vi "PID Controller.vi"() -> ()   [LabVIEW 2014]
panel:
  in  "Sample/sec":i32(slide) scale=0.0..50.0
  out "?":bool
  out "SP Vs PV":cluster{dbl, dbl}(knob)={0.0, 20.65645025147849} scale=0.0..60.0
  in  "?":bool
  in  "I":dbl=0.5
  in  "D":dbl=0.2
  in  "P":dbl=0.56
  in  "Minimum":dbl
  in  "Maximum":dbl=60.0
  in  "Set Point":dbl(slide)=50.0 scale=0.0..60.0
  out "Waveform Chart":cluster{"Set Point":dbl, "output variable":dbl}(graph)={"Set Point"=49.70711297071129, "output variable"=49.707112970712004}
  # "PID Temperature Controlller"
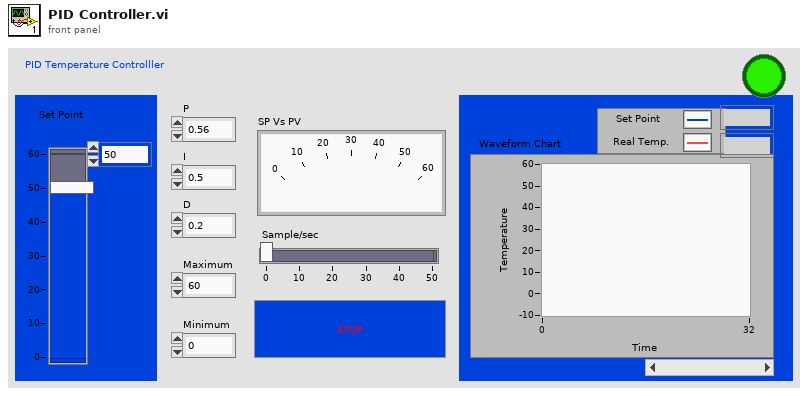
[diagram p1: front panel]
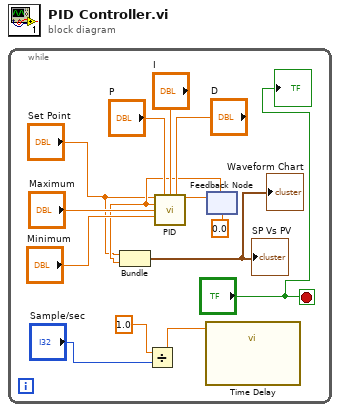
[diagram p0: block diagram]
diagram:
  n1 = while {
    stop <- "?" stop-if-true
    n2 = Divide(x=1.0, y="Sample/sec") -> (x/y=w1:dbl)
    n3 = call "Time Delay"("Delay Time (s)"=w1) -> ()  [unwired: 10 in, 1 out]
    n4 = feedback #1(0.0 ("output variable")) -> (w5:dbl)
    n5 = Bundle("Set Point"="Set Point", "output variable"=w5) -> (→"Waveform Chart" →"SP Vs PV":cluster{"Set Point":dbl, "output variable":dbl})  [unwired: 1 in]
    n6 = call "PID.vi"("sp"="Set Point", "p"="P", "i"="I", "d"="D", "pv"=w5, "maxim"="Maximum", "minim"="Minimum") -> ("output variable"=w9:dbl)  [unwired: 8 in]
    n7 = feedback-in #1(w9) -> ()
    "?" <- "?"
  }
